vi "Read preparePass.vi"(8 "error in (no error)":errorcluster, 11 "PassTactic in":refnum<class "PassTactic.lvclass">) -> (0 "error out":errorcluster, 2 "preparePass":bool, 3 "PassTactic out":refnum<class "PassTactic.lvclass">)   [LabVIEW 2023, in "PassTactic.lvclass"]
uses:
  PassTactic.lvclass
  PassTactic.lvclass/PassTactic.ctl
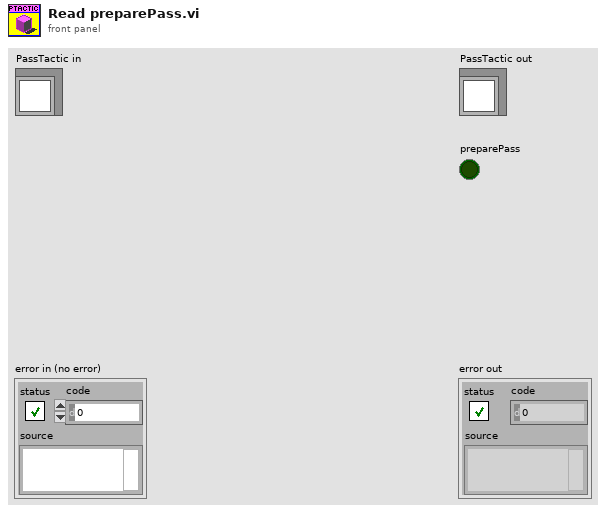
[diagram p1: front panel]
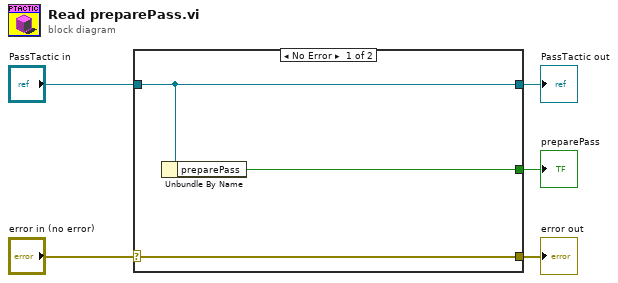
[diagram p0: block diagram]
diagram:
  n1 = case shown="No Error" "error in (no error)" {
    selector: "error in (no error)" -> [w8 w9]
    tunnel: [w8 w9] -> w4
    tunnel: [w7 w10] -> w2
    tunnel: "PassTactic in" -> [w7 w10]
    tunnel: [w6 _] -> w1
    frame No Error {
      n2 = Unbundle By Name(w7) -> ("preparePass"=w6:bool)
    }
    frame Error {
    }
  }
  "error out" <- w4
  "PassTactic out" <- w2
  "preparePass" <- w1
